vi "Wait for multiple events.vi"(8 "error in (no error)":errorcluster, 10 "Messages":string[](array[string]), 11 "Notifier in":refnum<notifier>) -> (0 "error out":errorcluster, 3 "Notifier out":refnum<notifier>)   [LabVIEW 2014]
panel:
  # "LICENSED MATERIALS – PROPERTY OF IBM\nCopyright IBM Corp. 2016,\nALL RIGHTS RESERVED"
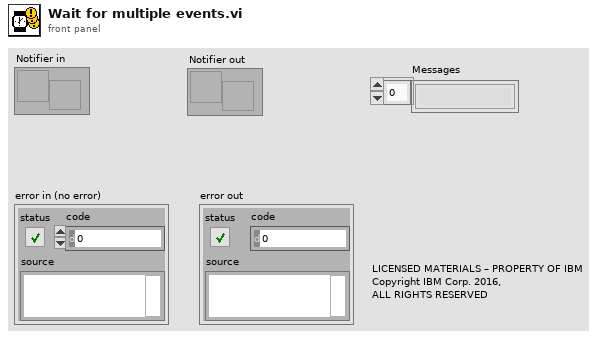
[diagram p1: front panel]
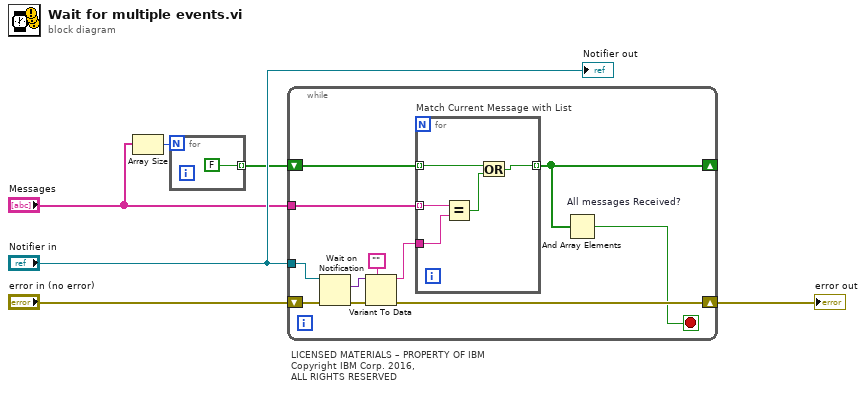
[diagram p0: block diagram]
diagram:
  # "LICENSED MATERIALS – PROPERTY OF IBM\nCopyright IBM Corp. 2016,\nALL RIGHTS RESERVED"
  n1 = Array Size(array="Messages") -> (size(s)=w3:i32)
  n2 = for {
    N: w3 -> [_]
    tunnel: [FALSE] -> w1 mode=indexing
  }
  n3 = while {
    shift-right: [w16] -> w6
    shift-left: "error in (no error)" -> [w18]
    tunnel: "Notifier in" -> [w13]
    tunnel: "Messages" -> [w12]
    shift-right: [w9] -> _
    shift-left: w1 -> [w11]
    stop <- w8 stop-if-true
    n4 = Wait on Notification(notifier=w13, error in (no error)=w18) -> (notification=w14:variant, error out=w17:errorcluster)  [unwired: 4 out]
    n5 = Variant To Data(error in=w17, type="", Variant=w14) -> (data=w10:string, error out=w16:errorcluster)
    n6 = for "Match Current Message with List" {
      tunnel: w12 -> [w23] mode=indexing
      tunnel: w11 -> [w21] mode=indexing
      tunnel: w10 -> [w22]
      tunnel: [w19] -> w9 mode=indexing
      n7 = Equal?(x=w23, y=w22) -> (x = y?=w20:bool)
      n8 = Or(x=w21, y=w20) -> (x .or. y?=w19:bool)
    }
    n9 = And Array Elements "All messages Received?"(Boolean array=w9) -> (logical AND=w8:bool)
  }
  "error out" <- w6
  "Notifier out" <- "Notifier in"
